vi "sv_UFF58 Check String.vi"(1 "operation":enum16{"read", "write"}(ring)=enum."write", 2 "use this string if field empty":string="NONE", 7 "field value":string, 13 "field length":i32=80) -> (8 "output string":string, 14 "is empty":bool)   [LabVIEW 2017, in "SoundVib_UFF58.lvlib"]
doc: "This VI checks if the input <B>field value</B> is empty. If empty it outputs the values in <B>use this string if field empty</B>. It also truncates the <B>field</B> if its length is greater than <B>field length</B>"
uses:
  <vilib>/addons/Sound and Vibration/svt_UFF58/SoundVib_UFF58.lvlib
  <vilib>/Utility/error.llb/whitespace.ctl
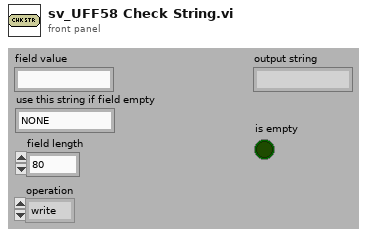
[diagram p1: front panel]
types:
  T1 = typedef "whitespace.ctl" = u16
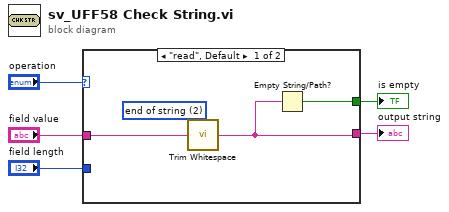
[diagram p0: block diagram]
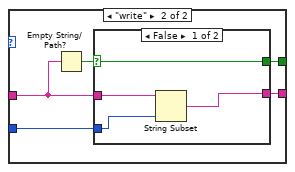
[diagram p2: hidden frame]
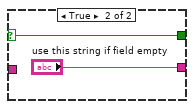
[diagram p3: hidden frame]
diagram:
  n1 = case shown="\"read\", Default" "operation" {
    tunnel: [w6 w14] -> w5
    tunnel: "field value" -> [w8 w13]
    tunnel: "field length" -> [_ w11]
    tunnel: [w7 w10] -> w2
    frame "read", Default {
      w9 = T1 2 items=["both", "start of string", "end of string"] ("location (both)")
      n2 = call <vilib>:"Trim Whitespace.vi"("string"=w8, "location (both)"=w9) -> ("trimmed string"=w6:string)
      n3 = Empty String/Path?(string/path=w6) -> (empty?=w7:bool)
    }
    frame "write" {
      n4 = Empty String/Path?(string/path=w13) -> (empty?=w12:bool)
      n5 = case shown="False" w12 {
        selector: w12 -> [w15 w19]
        tunnel: w13 -> [w17 _]
        tunnel: [w16 "use this string if field empty"] -> w14
        tunnel: w11 -> [w18 _]
        tunnel: [w15 w19] -> w10
        frame False {
          n6 = String Subset(string=w17, length (rest)=w18) -> (substring=w16:string)  [unwired: 1 in]
        }
        frame True {
        }
      }
    }
  }
  "output string" <- w5
  "is empty" <- w2
